vi "Power Spectrum (CDB).vi"(0 "X":cdb[](array[numeric])) -> (1 "Power Spectrum":dbl[](array[numeric]), 2 "error":i32)   [LabVIEW 2018, in "NI_AALPro.lvlib"]
doc: "Computes the <B>Power Spectrum</B>, Sxx, of the input sequence <B>X</B>. Wire data to the <B>X</B> input to determine the polymorphic instance to use or manually select the instance."
uses:
  NI_AALPro.lvlib
  <resource>/lvanlys.dll
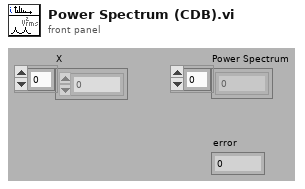
[diagram p1: front panel]
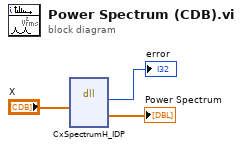
[diagram p0: block diagram]
diagram:
  n1 = dll-call lib="C:/Program Files (x86)/National Instruments/LabVIEW 2018/resource/lvanlys.*" fn="CxSpectrumH_IDP"("xH"="X") -> ("return type"=→"error":i32, "spectrumXH"=→"Power Spectrum":dbl[])  [unwired: 7 in, 2 out]
